vi "Write TDMS File Attributes.vi"(8 "error in (no error)":errorcluster, 10 "TDMS File Ref in":refnum<k34>, 11 "TDMS-Data in":refnum<class "TDMS-Data.lvclass">) -> (0 "error out":errorcluster, 2 "TDMS File Ref out":refnum<k34>, 3 "TDMS-Data out":refnum<class "TDMS-Data.lvclass">)   [LabVIEW 2016, in "BNT_TDMS.lvlib" / "TDMS-Data.lvclass"]
doc: "Write TDMS file attributes."
uses:
  TDMS-Data.lvclass
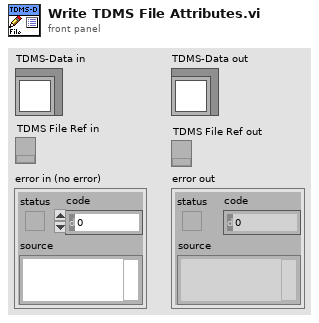
[diagram p1: front panel]
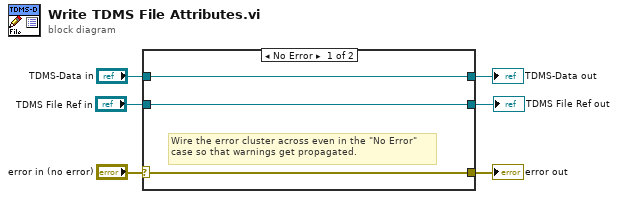
[diagram p0: block diagram]
diagram:
  n1 = case shown="No Error" "error in (no error)" {
    selector: "error in (no error)" -> [w8 w12]
    tunnel: [w8 w12] -> w5
    tunnel: [w9 w11] -> w3
    tunnel: "TDMS-Data in" -> [w9 w11]
    tunnel: [w7 w10] -> w2
    tunnel: "TDMS File Ref in" -> [w7 w10]
    frame No Error {
      # "Wire the error cluster across even in the \"No Error\"\ncase so that warnings get propagated."
    }
    frame Error {
    }
  }
  "error out" <- w5
  "TDMS-Data out" <- w3
  "TDMS File Ref out" <- w2
